vi "周期设置对话框.vi"() -> (2 "确定":bool, 3 "输出簇":T1)   [LabVIEW 2016]
uses:
  <vilib>/Utility/config.llb/Read Key (I32).vi
  <vilib>/Utility/config.llb/Read Key (Boolean).vi
  <vilib>/Utility/config.llb/Write Key (I32).vi
  <vilib>/Utility/config.llb/Write Key (Boolean).vi
  <vilib>/Utility/config.llb/NI_LVConfig.lvlib
panel:
  in  "氨氮":bool
  in  "CODCr":bool
  in  "多参数":bool
  in  "运行模式":enum16{"维护模式", "常规模式", "应急模式", "质控模式"}(ring)
  in  "运行间隔":i16=4 min=1 max=24
  in  "取消":bool
  in  "确定":bool
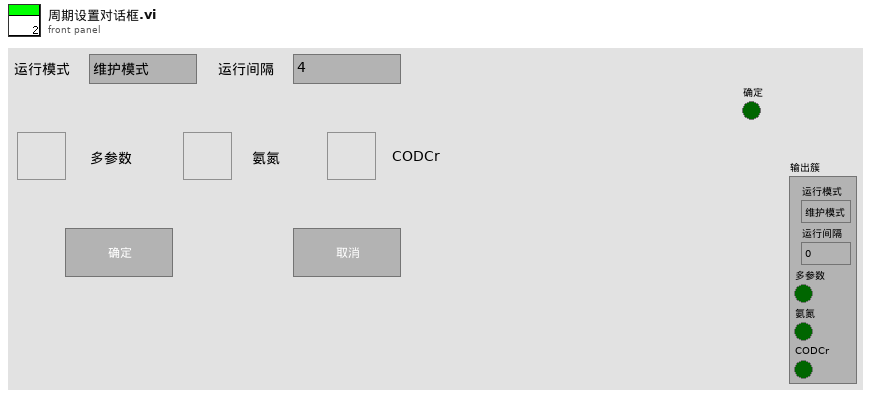
[diagram p1: front panel]
types:
  T1 = cluster{"运行模式":enum16{"维护模式", "常规模式", "应急模式", "质控模式"}, "运行间隔":i16, "多参数":bool, "氨氮":bool, "CODCr":bool}
  T2 = typedef "NI_LVConfig.lvlib/Config Data RefNum.ctl" = refnum<k1>
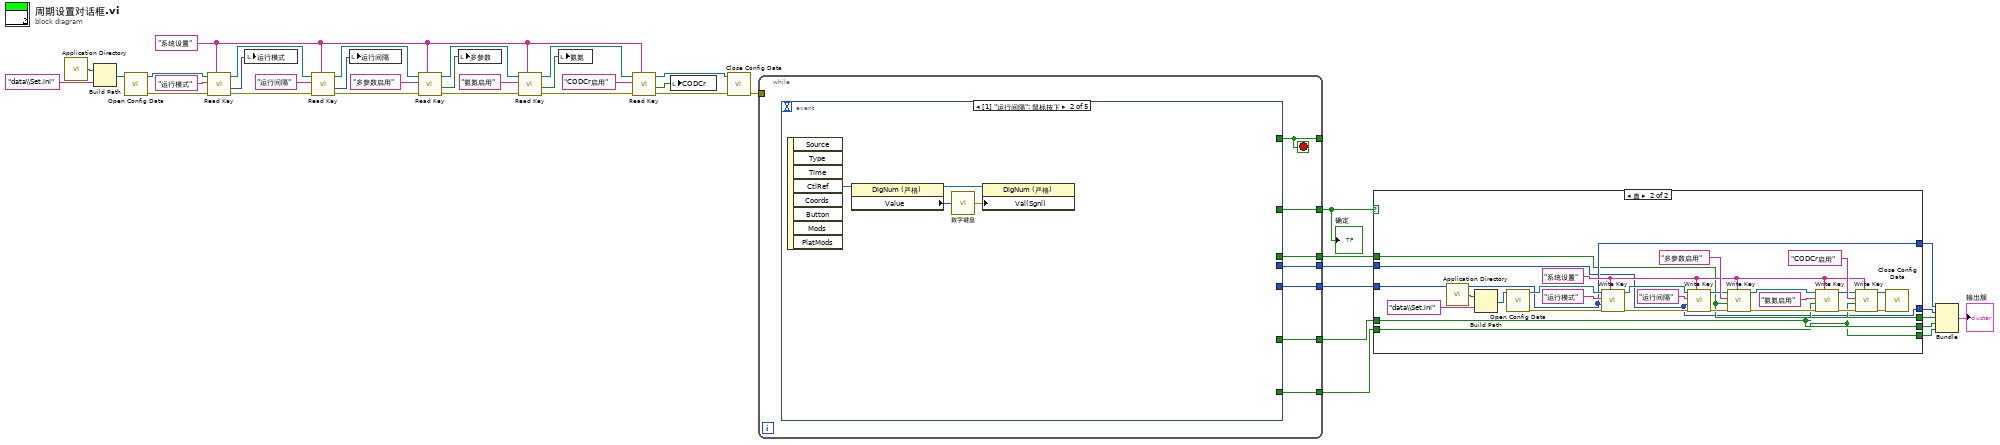
[diagram p0: block diagram]
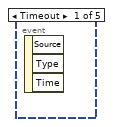
[diagram p3: hidden frame]
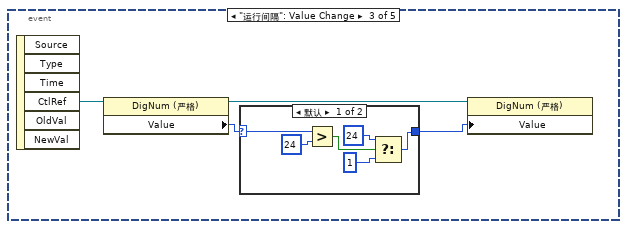
[diagram p4: hidden frame]
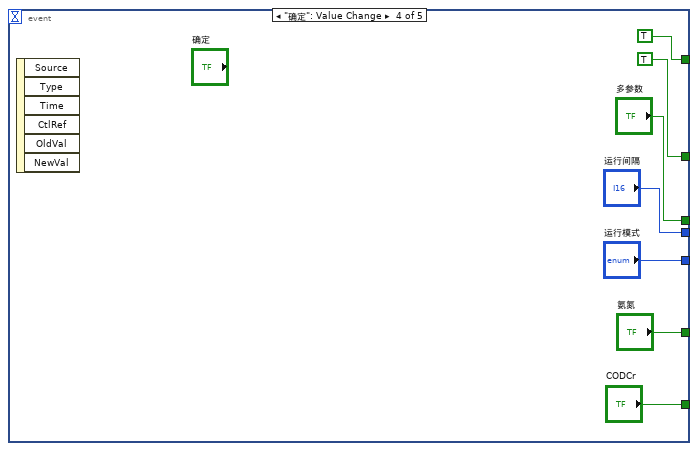
[diagram p6: hidden frame]
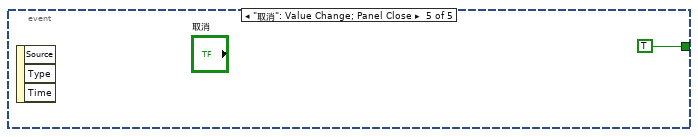
[diagram p7: hidden frame]
diagram:
  w24 = "系统设置" ("section")
  n1 = call <vilib>:"Application Directory.vi"() -> ("Application Directory"=w9:path)
  n2 = Build Path(base path=w9, name or relative path="data\\Set.ini" ("名称或相对路径")) -> (appended path=w11:path)
  n3 = call <vilib>:"Open Config Data.vi"("configuration file path"=w11) -> ("error out"=w8:errorcluster, "refnum"=w7:T2)  [unwired: 8 in, 1 out]
  n4 = call-poly <vilib>:"Read Key.vi"("section"=w24, "error in (no error)"=w8, "key"="运行模式" ("section"), "refnum"=w7) -> ("error out"=w13:errorcluster, "value"=w6:i32, "refnum out"=w12:T2)  [unwired: 4 in, 1 out]
  n5 = local write "运行模式"(w6) -> ()
  n6 = call-poly <vilib>:"Read Key.vi"("section"=w24, "error in (no error)"=w13, "key"="运行间隔" ("section"), "refnum"=w12) -> ("error out"=w20:errorcluster, "value"=w5:i32, "refnum out"=w18:T2)  [unwired: 4 in, 1 out]
  n7 = local write "运行间隔"(w5) -> ()
  n8 = call-poly <vilib>:"Read Key.vi"("section"=w24, "error in (no error)"=w20, "key"="多参数启用" ("section"), "refnum"=w18) -> ("error out"=w16:errorcluster, "value"=w4:bool, "refnum out"=w17:T2)  [unwired: 4 in, 1 out]
  n9 = local write "多参数"(w4) -> ()
  n10 = call-poly <vilib>:"Read Key.vi"("section"=w24, "error in (no error)"=w16, "key"="氨氮启用" ("section"), "refnum"=w17) -> ("error out"=w21:errorcluster, "value"=w3:bool, "refnum out"=w19:T2)  [unwired: 4 in, 1 out]
  n11 = local write "氨氮"(w3) -> ()
  n12 = call-poly <vilib>:"Read Key.vi"("section"=w24, "error in (no error)"=w21, "key"="CODCr启用" ("section"), "refnum"=w19) -> ("error out"=w22:errorcluster, "value"=w2:bool, "refnum out"=w23:T2)  [unwired: 4 in, 1 out]
  n13 = local write "CODCr"(w2) -> ()
  n14 = call <vilib>:"Close Config Data.vi"("error in (no error)"=w22, "refnum"=w23) -> ("error out"=w1:errorcluster)  [unwired: 8 in, 1 out]
  n15 = while {
    tunnel: [w46] -> _
    tunnel: [w45] -> w39
    tunnel: [w44] -> w36
    tunnel: [w43] -> w35
    tunnel: [w42] -> w34
    tunnel: [w41] -> w37
    tunnel: [w40] -> w38
    tunnel: w1 -> [_]
    stop <- w46 stop-if-true
    n16 = event shown="[1] \"运行间隔\": 鼠标按下" {
      selector: _ -> [_ _ _ _ _]
      dyn-events: _ -> [_ _ _ _ _]
      timeout: _ -> [_ _ _ _ _]
      tunnel: [_ _ _ TRUE TRUE] -> w46
      tunnel: [_ _ _ TRUE _] -> w45
      tunnel: [_ _ _ "多参数" _] -> w44
      tunnel: [_ _ _ "氨氮" _] -> w43
      tunnel: [_ _ _ "CODCr" _] -> w42
      tunnel: [_ _ _ "运行模式" _] -> w41
      tunnel: [_ _ _ "运行间隔" _] -> w40
      event Timeout {
        n17 = event-data() -> ()  [unwired: 1 in, 3 out]
      }
      event "运行间隔": Mouse Down {
        n18 = event-data() -> ("CtlRef"=w47:refnum<vi>)  [unwired: 1 in, 7 out]
        n19 = property class="DigNum (严格)"(reference=w47) -> (reference out=w49:refnum<vi>, "Value"=w50:i16)  [unwired: 1 in, 1 out]
        n20 = call "数字键盘.vi"("OldNumber"=w50) -> ("NewNumber"=w48:sgl)
        n21 = property class="DigNum (严格)"(reference=w49, "Val(Sgnl)"=w48) -> ()  [unwired: 1 in, 2 out]
      }
      event "运行间隔": Value Change {
        n22 = event-data() -> ("CtlRef"=w54:refnum<vi>)  [unwired: 1 in, 5 out]
        n23 = property class="DigNum (严格)"(reference=w54) -> (reference out=w52:refnum<vi>, "Value"=w53:i16)  [unwired: 1 in, 1 out]
        n24 = case shown="默认" w53 {
          selector: w53 -> [w57 w61]
          tunnel: [w56 w61] -> w51
          frame Default {
            n25 = Greater?(x=w57, y=i16 24) -> (0:w59:bool)
            n26 = Select(t=i16 24 ("y"), s=w59, f=i16 1) -> (s? t:f=w56:i16)
          }
          frame 1..24 {
          }
        }
        n27 = property class="DigNum (严格)"(reference=w52, "Value"=w51) -> ()  [unwired: 1 in, 2 out]
      }
      event "确定": Value Change {
        n28 = event-data() -> ()  [unwired: 1 in, 6 out]
      }
      event "取消": Value Change; Panel Close {
        n29 = event-data() -> ()  [unwired: 1 in, 3 out]
      }
    }
  }
  "确定" <- w39
  n30 = case shown="真" w39 {
    tunnel: w38 -> [_ w70]
    tunnel: w37 -> [_ w74]
    tunnel: w36 -> [_ w73]
    tunnel: w35 -> [_ w72]
    tunnel: w34 -> [_ w71]
    tunnel: [_ w74] -> w33
    tunnel: [_ w70] -> w32
    tunnel: [_ w73] -> w31
    tunnel: [_ w72] -> w30
    tunnel: [_ w71] -> w29
    frame False {
    }
    frame True {
      w92 = "系统设置" ("section")
      n31 = call <vilib>:"Application Directory.vi"() -> ("Application Directory"=w77:path)
      n32 = Build Path(base path=w77, name or relative path="data\\Set.ini" ("名称或相对路径")) -> (appended path=w79:path)
      n33 = call <vilib>:"Open Config Data.vi"("configuration file path"=w79) -> ("error out"=w76:errorcluster, "refnum"=w75:T2)  [unwired: 8 in, 1 out]
      n34 = call-poly <vilib>:"Write Key.vi"("section"=w92, "error in (no error)"=w76, "value"=w74, "key"="运行模式" ("section"), "refnum"=w75) -> ("error out"=w81:errorcluster, "refnum out"=w80:T2)  [unwired: 4 in, 1 out]
      n35 = call-poly <vilib>:"Write Key.vi"("section"=w92, "error in (no error)"=w81, "value"=w70, "key"="运行间隔" ("section"), "refnum"=w80) -> ("error out"=w88:errorcluster, "refnum out"=w86:T2)  [unwired: 4 in, 1 out]
      n36 = call-poly <vilib>:"Write Key.vi"("section"=w92, "error in (no error)"=w88, "value"=w73, "key"="多参数启用" ("section"), "refnum"=w86) -> ("error out"=w84:errorcluster, "refnum out"=w85:T2)  [unwired: 4 in, 1 out]
      n37 = call-poly <vilib>:"Write Key.vi"("section"=w92, "error in (no error)"=w84, "value"=w72, "key"="氨氮启用" ("section"), "refnum"=w85) -> ("error out"=w89:errorcluster, "refnum out"=w87:T2)  [unwired: 4 in, 1 out]
      n38 = call-poly <vilib>:"Write Key.vi"("section"=w92, "error in (no error)"=w89, "value"=w71, "key"="CODCr启用" ("section"), "refnum"=w87) -> ("error out"=w90:errorcluster, "refnum out"=w91:T2)  [unwired: 4 in, 1 out]
      n39 = call <vilib>:"Close Config Data.vi"("error in (no error)"=w90, "refnum"=w91) -> ()  [unwired: 8 in, 2 out]
    }
  }
  n40 = Bundle("运行模式"=w33, "运行间隔"=w32, "多参数"=w31, "氨氮"=w30, "CODCr"=w29) -> (→"输出簇":T1)  [unwired: 1 in]
